vi "RT_MasterLoop_JointAngle.vi"   [LabVIEW 2016]
uses:
  Shared Libraries/VN100/TypeDef/AsyncMode.ctl
  Remote VIs/Configs/CMSMismatch.ctl
  Classes/CAlex2/TypeDef/CAlexVersion.ctl
  <vilib>/FPGAPlugInAG/PXI-7842R/niLvFpga_Open_PXI-7842R.vi
  <vilib>/rvi/interface/common/dynamic/niFpgaDynamicAddResources.vi
  <vilib>/rvi/interface/nirviOpenFPGA/nirviOpenFPGA.xnode
  FPGA Bitfiles/CAlex2_FPGATarget_MotorControl_+dy1qhm6Ymw.lvbitx
  Shared Libraries/VN100/VN100.lvclass
  Classes/CAlex2/CAlex2.lvclass
  <vilib>/AuZn/auzn custom VIs/AuZnCustomVI.lvlib
panel:
  # "Angles Version"
  # "This VI can only be stopped by pressing the stop button on the control interface VI"
types:
  T1 = typedef "CMSMismatch.ctl" = cluster{"TotalCount":cluster{"CableCount":i32, "MotorCount":i32, "SensorCount":i32}, "Matches":cluster{"CableID":i32, "MotorID":i32, "SensorID":i32}[]}
  T2 = typedef "VN100.lvclass/AsyncMode.ctl" = enum16{"VNYPR", "VNYMR"}
  T3 = typedef "CAlex2.lvclass/CAlexVersion.ctl" = enum16{"Bilateral_Squat", "Squat", "Treadmill", "Mobile"}
  T4 = typedef "LowLvControl Cluster.ctl" = cluster{"MotorCtrl":refnum<class "MotorControl.lvclass">, "FPGA Ref":refnum<k20>, "AI Task":refnum<k21>, "Encoder Tasks":refnum<k21>[]}
  T5 = typedef "HighLvControl Cluster.ctl" = cluster{"CAlexVersion":T3, "CAlex2 out":refnum<class "CAlex2.lvclass">, "ForceField":refnum<class "ForceField.lvclass">}
  T6 = typedef "Logger Cluster.ctl" = cluster{"Data Logger out":refnum<class "Data Logger.lvclass">, "CAlexVersion":T3, "SyncIn":refnum<k21>, "SyncOut":refnum<k21>}
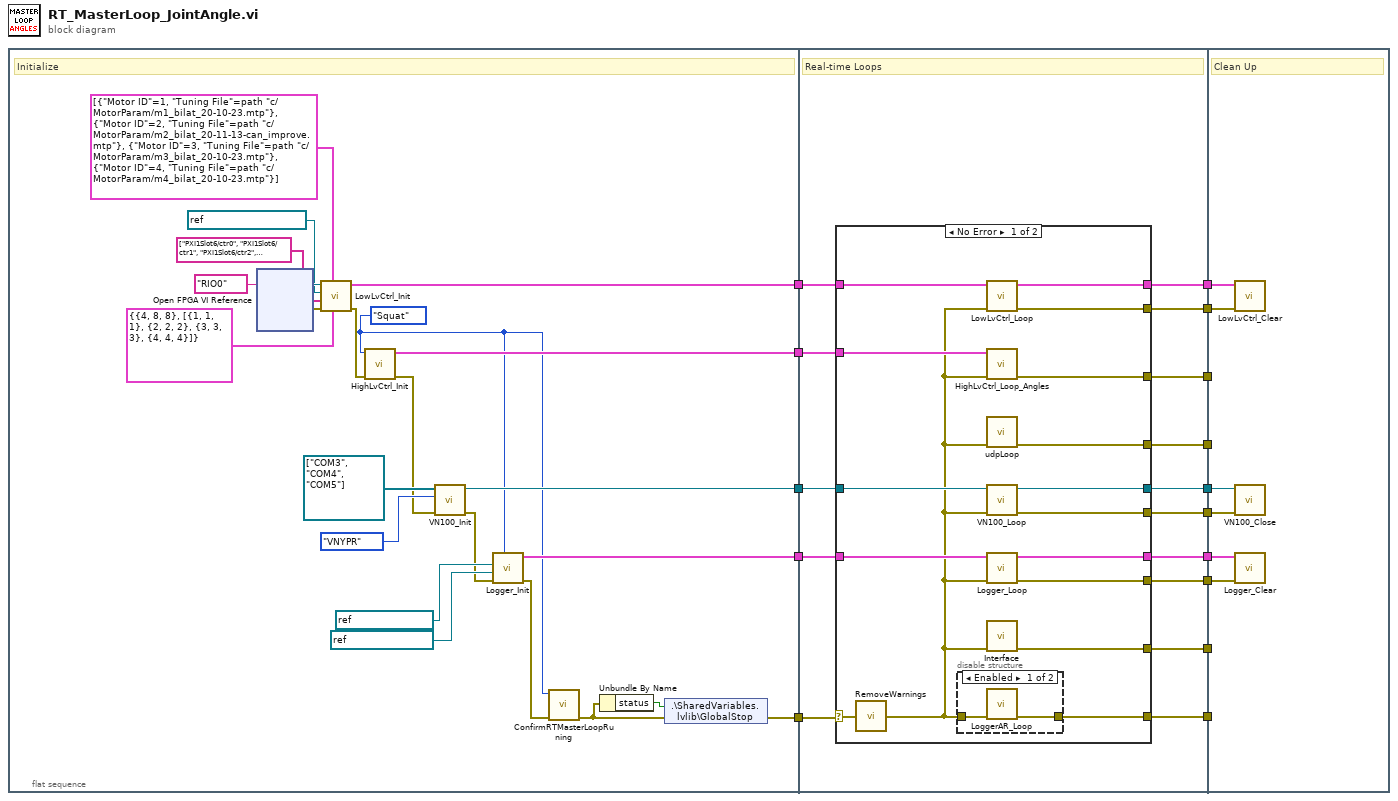
[diagram p0: block diagram]
diagram:
  n1 = flat-sequence {
    tunnel: [w33] -> w15
    tunnel: [w38] -> w14
    tunnel: [w37] -> w10
    tunnel: [w35] -> w9
    tunnel: [w34] -> w8
    tunnel: w15 -> [w53]
    tunnel: w14 -> [w52]
    tunnel: [w51] -> w13
    tunnel: [w50] -> w12
    tunnel: [w49] -> w11
    tunnel: w10 -> [w48]
    tunnel: w9 -> [w47]
    tunnel: w8 -> [w46]
    tunnel: [w45] -> w7
    tunnel: [w44] -> w6
    tunnel: [w43] -> w5
    tunnel: [w42] -> w4
    tunnel: [w41] -> w3
    tunnel: [w40] -> w2
    tunnel: [w39] -> w1
    tunnel: w13 -> [w81]
    tunnel: w12 -> [w80]
    tunnel: w11 -> [_]
    tunnel: w7 -> [w77]
    tunnel: w6 -> [w79]
    tunnel: w5 -> [w78]
    tunnel: w4 -> [w76]
    tunnel: w3 -> [_]
    tunnel: w2 -> [_]
    tunnel: w1 -> [_]
    frame #0 {
      w16 = CAlexVersion."Squat" ("CAlexVersion")
      # "Initialize"
      n2 = xnode "Open FPGA VI Reference"("resource name"=tag "RIO0") -> ("FPGA VI Reference Out"=w23:refnum<k20>, "error out"=w30:errorcluster)  [unwired: 1 in]
      n3 = call "LowLvCtrl_Init.vi"("CMSMismatch"=T1 {"TotalCount"={"CableCount"=4, "MotorCount"=8, "SensorCount"=8}, "Matches"=[{"CableID"=1, "MotorID"=1, "SensorID"=1}, {"CableID"=2, "MotorID"=2, "SensorID"=2}, {"CableID"=3, "MotorID"=3, "SensorID"=3}, {"CableID"=4, "MotorID"=4, "SensorID"=4}]}, "MTP Files"=cluster{"Motor ID":i32, "Tuning File":path}[] [{"Motor ID"=1, "Tuning File"=path "c:/MotorParam/m1_bilat_20-10-23.mtp"}, {"Motor ID"=2, "Tuning File"=path "c:/MotorParam/m2_bilat_20-11-13-can_improve.mtp"}, {"Motor ID"=3, "Tuning File"=path "c:/MotorParam/m3_bilat_20-10-23.mtp"}, {"Motor ID"=4, "Tuning File"=path "c:/MotorParam/m4_bilat_20-10-23.mtp"}], "error in (no error)"=w30, "Encoder Tasks In"=tag[] ["PXI1Slot6/ctr0", "PXI1Slot6/ctr1", "PXI1Slot6/ctr2", "PXI1Slot6/ctr3", "PXI1Slot6/ctr4", "PXI1Slot6/ctr5", "PXI1Slot6/ctr6", "PXI1Slot6/ctr7"], "Analog Task In"=refnum<k21> "LoadCells_FSR_AI", "FPGA VI Reference In"=w23) -> ("error out"=w32:errorcluster, "LowLvControl"=w33:T4)  [unwired: 4 in]
      n4 = call "HighLvCtrl_Init.vi"("error in (no error)"=w32, "CAlexVersion"=w16) -> ("error out"=w24:errorcluster, "HighLvClasses"=w38:T5)  [unwired: 8 in]
      n5 = call "VN100_Init.vi"("error in (no error)"=w24, "AsyncMode(VNYPR)"=AsyncMode."VNYPR" ("AsyncMode"), "Serial Ports"=refnum<visa-resource-name>[] ["COM3", "COM4", "COM5"]) -> ("error out"=w26:errorcluster, "VN100 out"=w35:refnum<class "VN100.lvclass">)  [unwired: 7 in]
      n6 = call "Logger_Init.vi"("CAlexVersion"=w16, "error in (no error)"=w26, "SyncOut"=refnum<k21> "SyncOut_EMG" ("SyncOut_EMG"), "SyncIn"=refnum<k21> "SyncIn_Vicon" ("SyncOut_EMG")) -> ("error out"=w18:errorcluster, "Logger Loop Cluster"=w34:T6)  [unwired: 6 in]
      n7 = call "ConfirmRTMasterLoopRuning.vi"("error in (no error)"=w18, "CAlexVersion"=w16) -> ("error out"=w17:errorcluster)  [unwired: 9 in]
      n8 = Unbundle By Name(w17) -> ("status"=w36:bool)
      n9 = shared-variable ".\\SharedVariables.lvlib\\GlobalStop"(w36, error in=w17) -> (error out=w37:errorcluster)
    }
    frame #1 {
      # "Real-time Loops"
      n10 = case shown="No Error" w48 {
        selector: w48 -> [w59 w72]
        tunnel: w53 -> [w62 w74]
        tunnel: w52 -> [w65 _]
        tunnel: [w69 w75] -> w51
        tunnel: [w68 w72] -> w50
        tunnel: [w67 w72] -> w49
        tunnel: w47 -> [w66 w75]
        tunnel: [w64 w72] -> w45
        tunnel: w46 -> [w63 w73]
        tunnel: [w61 w74] -> w44
        tunnel: [w60 w72] -> w43
        tunnel: [w58 w73] -> w42
        tunnel: [w57 w72] -> w41
        tunnel: [w56 w72] -> w40
        tunnel: [w55 w72] -> w39
        frame No Error {
          n11 = call <vilib>:"RemoveWarnings.vi"("error in (no error)"=w59) -> ("error out"=w54:errorcluster)
          n12 = disable-structure shown="Enabled" {
            disable-tunnel: w54 -> [w71 _]
            disable-tunnel: [w70 _] -> w55
            frame Enabled {
              n13 = call "LoggerAR_Loop.vi"("error in (no error)"=w71) -> ("error out"=w70:errorcluster)  [unwired: 10 in]
            }
            frame Disabled {
            }
          }
          n14 = call "LowLvCtrl_Loop.vi"("error in (no error)"=w54, "LowLvControl in"=w62) -> ("error out"=w60:errorcluster, "LowLvControl out"=w61:T4)  [unwired: 8 in]
          n15 = call "HighLvCtrl_Loop_Angles.vi"("error in (no error)"=w54, "HighLvClasses"=w65) -> ("error out"=w57:errorcluster)  [unwired: 9 in]
          n16 = call "udpLoop.vi"("error in (no error)"=w54) -> ("error out"=w56:errorcluster)  [unwired: 10 in]
          n17 = call "VN100_Loop.vi"("error in (no error)"=w54, "VN100 In"=w66) -> ("error out"=w68:errorcluster, "VN100 Out"=w69:refnum<class "VN100.lvclass">)  [unwired: 8 in]
          n18 = call "Logger_Loop.vi"("error in (no error)"=w54, "Logger Loop Cluster in"=w63) -> ("error out"=w64:errorcluster, "Logger Cluster out"=w58:T6)  [unwired: 8 in]
          n19 = call "Interface.vi"("error in (no error)"=w54) -> ("error out"=w67:errorcluster)  [unwired: 10 in]
        }
        frame Error {
        }
      }
    }
    frame #2 {
      # "Clean Up"
      n20 = call "LowLvCtrl_Clear.vi"("error in (no error)"=w78, "LowLvControl"=w79) -> ()  [unwired: 9 in, 1 out]
      n21 = call "VN100_Close.vi"("error in (no error)"=w80, "VN100 in"=w81) -> ()  [unwired: 9 in, 1 out]
      n22 = call "Logger_Clear.vi"("error in (no error)"=w77, "Logger Loop Cluster"=w76) -> ()  [unwired: 9 in, 1 out]
    }
  }
